vi "Get Minimum Log Level.vi"(8 "error in (no error)":errorcluster, 11 "logger name":string) -> (0 "error out":errorcluster, 3 "minimum log level":T1)   [LabVIEW 2018, in "GLog.lvlib" / "Registry.lvlib"]
uses:
  Registry.lvlib
  api/Log Levels.ctl
  Registry Actions.ctl
  dependencies/Utilities/Utilities.lvlib
  api/GLog.lvlib
panel:
  # "Connector Pane"
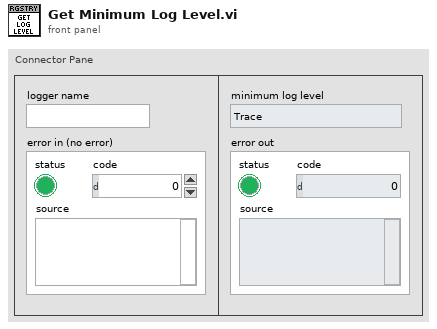
[diagram p1: front panel]
types:
  T1 = typedef "GLog.lvlib/Log Levels.ctl" = enum16{"Trace", "Debug", "Info", "Warning", "Error", "Critical"}
  T2 = cluster{"log level":T1, "error out":errorcluster}
  T3 = typedef "GLog.lvlib/Registry.lvlib/Registry Actions.ctl" = enum16{"Register", "Log", "Enable", "Enable All", "Disable", "Disable All", "Get Enable State", "Get Minimum Log Level", "Set Minimum Log Level", "Set All Minimum Log Level", "Get Logger Info", "Get All Logger Info", "List", "Unregister", "Unregister All", "Shutdown"}
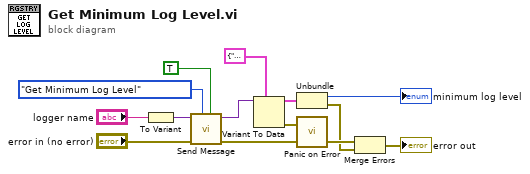
[diagram p0: block diagram]
diagram:
  n1 = To Variant(anything="logger name") -> (Variant=w10:variant)
  n2 = call "Send Message.vi"("return data? (F)"=TRUE, "action"=Registry_Actions."Get Minimum Log Level", "error in (no error)"="error in (no error)", "send data"=w10) -> ("error out"=w13:errorcluster, "return data"=w8:variant)  [unwired: 6 in]
  n3 = Variant To Data(type=T2 {"log level"=enum."Trace", "error out"={"status"=FALSE, "code"=0, "source"=""}}, Variant=w8) -> (data=w3:T2, error out=w7:errorcluster)  [unwired: 1 in]
  n4 = Unbundle(w3) -> ("log level"=→"minimum log level":T1, "error out"=w2:errorcluster)
  n5 = call "Panic on Error.vi"("error in (no error)"=w7) -> ()  [unwired: 3 in]
  n6 = Merge Errors(w13, w2) -> (→"error out":errorcluster)
